vi "ReadM2VelocityPID.vi"(8 "error in (no error)":errorcluster, 11 "VISA Refnum in":refnum<visa-resource-name>) -> (0 "error out":errorcluster, 2 "Valid":bool, 3 "VISA Refnum out":refnum<visa-resource-name>, 4 "QPPS":u32, 5 "Ki":u32, 6 "Kd":u32, 7 "Kp":u32)   [LabVIEW 2015, in "Ion Motion Roboclaw.lvlib"]
uses:
  <instrlib>/Ion Motion Roboclaw/Ion Motion Roboclaw.lvlib
panel:
  in  "Address":u8
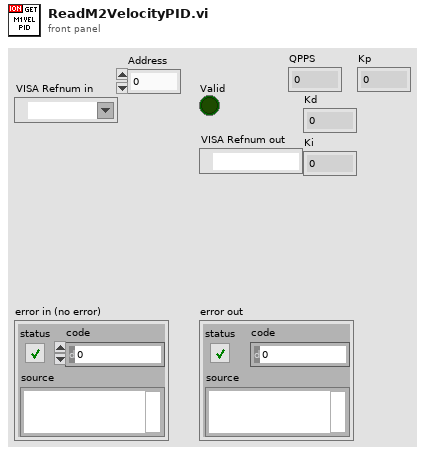
[diagram p1: front panel]
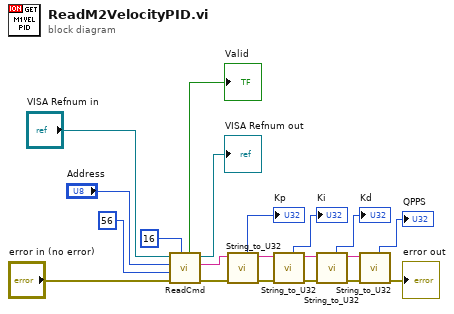
[diagram p0: block diagram]
diagram:
  n1 = call <instrlib>:"ReadCmd.vi"("Read Count"=u32 16, "error in (no error)"="error in (no error)", "Cmd"=u8 56, "Address"="Address", "VISA Refnum in"="VISA Refnum in") -> ("error out"=w7:errorcluster, "Output"=w8:string, "VISA Refnum out"=→"VISA Refnum out":refnum<visa-resource-name>, "Valid"=→"Valid":bool)  [unwired: 3 in]
  n2 = call <instrlib>:"String_to_U32.vi"("error in (no error)"=w7, "String"=w8) -> ("error out"=w17:errorcluster, "rest of the binary string"=w20:string, "number"=→"Kp":u32)  [unwired: 5 in]
  n3 = call <instrlib>:"String_to_U32.vi"("error in (no error)"=w17, "String"=w20) -> ("error out"=w16:errorcluster, "rest of the binary string"=w19:string, "number"=→"Ki":u32)  [unwired: 5 in]
  n4 = call <instrlib>:"String_to_U32.vi"("error in (no error)"=w16, "String"=w19) -> ("error out"=w15:errorcluster, "rest of the binary string"=w18:string, "number"=→"Kd":u32)  [unwired: 5 in]
  n5 = call <instrlib>:"String_to_U32.vi"("error in (no error)"=w15, "String"=w18) -> ("error out"=→"error out":errorcluster, "number"=→"QPPS":u32)  [unwired: 5 in, 1 out]
